vi "chat.vi"() -> ()   [LabVIEW 2016]
uses:
  <vilib>/httpClient/POSTBuffer.vi
  <vilib>/httpClient/LabVIEWHTTPClient.lvlib
panel:
  out "Error Msg":string
  out "OK?":bool
  out "Reply":string
  in  "Agent ID":string
  in  "User Text":string
  out "error out":errorcluster
  in  "error in":errorcluster
  in  "Base URL":string="http://localhost:3000"
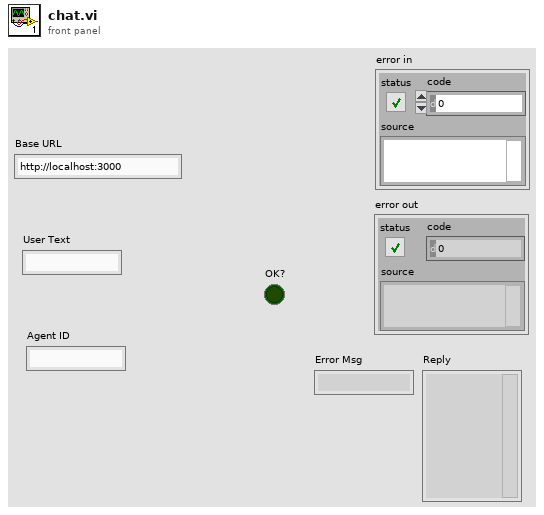
[diagram p1: front panel]
types:
  T1 = cluster{"ok":bool, "reply":string, "agentId":string, "agentName":string, "model":string, "error":string}
  T2 = typedef "LabVIEWHTTPClient.lvlib/ClientHandle.ctl" = refnum<k1>
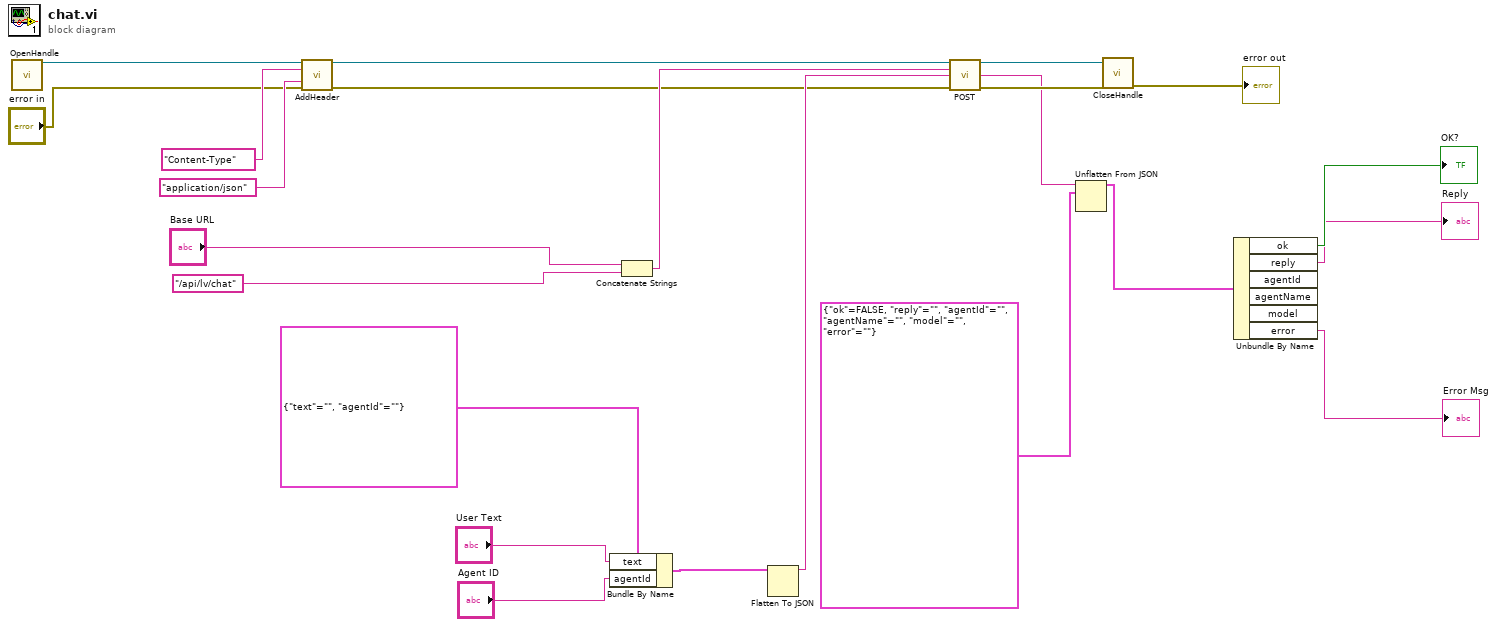
[diagram p0: block diagram]
diagram:
  n1 = call <vilib>:"OpenHandle.vi"() -> ("client handle out"=w21:T2)  [unwired: 14 in, 1 out]
  n2 = call <vilib>:"AddHeader.vi"("client handle"=w21, "header"="Content-Type", "value"="application/json", "error in (no error)"="error in") -> ("client handle out"=w18:T2, "error out"=w9:errorcluster)  [unwired: 10 in]
  n3 = Bundle By Name(cluster=cluster{"text":string, "agentId":string} {"text"="", "agentId"=""}, "text"="User Text", "agentId"="Agent ID") -> (w13:cluster{"text":string, "agentId":string})
  n4 = Concatenate Strings("Base URL", "/api/lv/chat") -> (w17:string)
  n5 = Flatten To JSON(anything=w13) -> (JSON string=w12:string)  [unwired: 2 in, 1 out]
  n6 = call-poly <vilib>:"POST.vi"("client handle"=w18, "url"=w17, "buffer"=w12, "error in (no error)"=w9) -> ("client handle out"=w11:T2, "body"=w7:string, "error out"=w8:errorcluster)  [unwired: 8 in, 1 out]
  n7 = Unflatten From JSON(JSON string=w7, type and defaults=T1 {"ok"=FALSE, "reply"="", "agentId"="", "agentName"="", "model"="", "error"=""}) -> (value=w5:T1)  [unwired: 5 in, 1 out]
  n8 = call <vilib>:"CloseHandle.vi"("client handle"=w11, "error in (no error)"=w8) -> ("error out"=→"error out":errorcluster)  [unwired: 13 in]
  n9 = Unbundle By Name(w5) -> ("ok"=→"OK?":bool, "reply"=→"Reply":string, "error"=→"Error Msg":string)  [unwired: 3 out]
